vi "constructor.vi"(10 "col":u8, 11 "row":u8) -> (3 "field":refnum<class "BoardField.lvclass">)   [LabVIEW 2017, in "BoardField.lvclass"]
uses:
  BoardField.lvclass
  BoardField.lvclass/BoardField.ctl
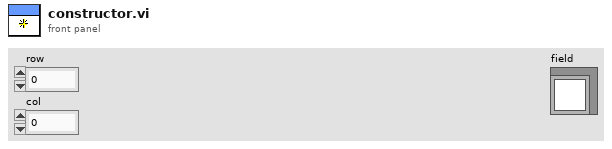
[diagram p1: front panel]
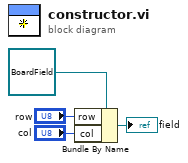
[diagram p0: block diagram]
diagram:
  n1 = Bundle By Name(cluster=refnum<class "BoardField.lvclass"> refnum ("BoardField.lvclass"), "row"="row", "col"="col") -> (→"field":refnum<class "BoardField.lvclass">)
